vi "subConvertValueToNameAndPath.vi"(9 "Project path":path, 11 "Value":string) -> (1 "Path":path, 3 "Name":string)   [LabVIEW 2020, in "SolutionBuilder.lvlib"]
uses:
  SolutionBuilder.lvlib
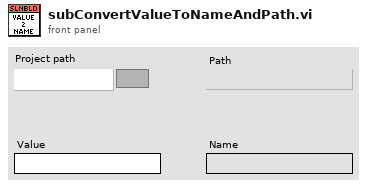
[diagram p1: front panel]
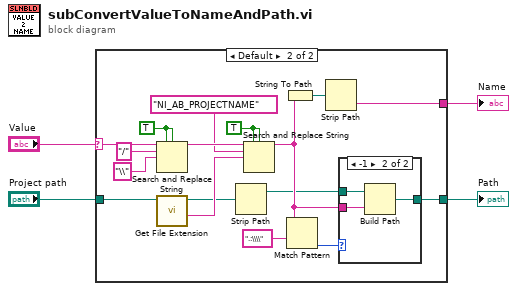
[diagram p0: block diagram]
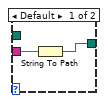
[diagram p3: hidden frame]
diagram:
  n1 = case shown="Default" "Value" {
    selector: "Value" -> [_ w6]
    tunnel: [_ w14] -> w1
    tunnel: "Project path" -> [_ w13]
    tunnel: [_ w7] -> w3
    frame "" {
    }
    frame Default {
      w18 = TRUE ("replace all? (F)")
      w19 = TRUE ("replace all? (F)")
      n2 = Search and Replace String(replace all?=w19, case sensitive?=w19, input string=w6, search string="/", replace string="\\" ("replace string (\"\")")) -> (result string=w17:string)  [unwired: 3 in, 3 out]
      n3 = call <vilib>:"Get File Extension.vi"("file"=w13) -> ("filename without extension"=w12:string, "dup file"=w9:path)  [unwired: 6 in, 3 out]
      n4 = Strip Path(path=w9) -> (stripped path=w5:path)  [unwired: 1 out]
      n5 = Search and Replace String(replace all?=w18, case sensitive?=w18, input string=w17, search string="NI_AB_PROJECTNAME", replace string=w12) -> (result string=w8:string)  [unwired: 3 in, 3 out]
      n6 = String To Path(string=w8) -> (path=w15:path)
      n7 = Match Pattern(string=w8, regular expression=".:\\\\") -> (offset past match=w10:i32)  [unwired: 1 in, 3 out]
      n8 = Strip Path(path=w15) -> (name=w14:string)  [unwired: 1 out]
      n9 = case shown="-1" w10 {
        tunnel: w5 -> [_ w26]
        tunnel: w8 -> [w23 w25]
        tunnel: [w22 w24] -> w7
        frame Default {
          n10 = String To Path(string=w23) -> (path=w22:path)
        }
        frame -1 {
          n11 = Build Path(base path=w26, name or relative path=w25) -> (appended path=w24:path)
        }
      }
    }
  }
  "Path" <- w3
  "Name" <- w1
